vi "sequence1.vi"() -> ()   [LabVIEW 2021]
panel:
  out "Array":i64[](array[numeric])
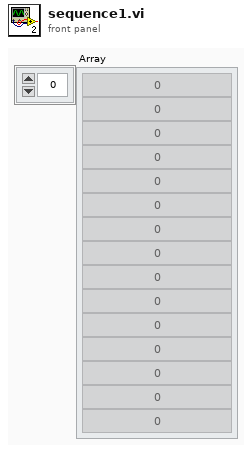
[diagram p1: front panel]
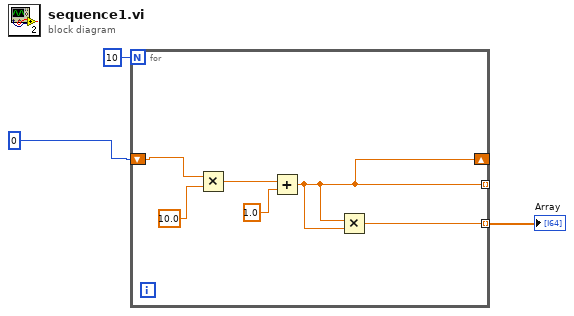
[diagram p0: block diagram]
diagram:
  n1 = for {
    N: 10 -> [_]
    shift-right: [w4] -> _
    shift-left: 0 -> [w8]
    tunnel: [w4] -> _ mode=indexing
    tunnel: [w6] -> w2 mode=indexing
    n2 = Multiply(x=w8, y=10.0) -> (x*y=w5:dbl)
    n3 = Add(x=w5, y=1.0) -> (x+y=w4:dbl)
    n4 = Multiply(x=w4, y=w4) -> (x*y=w6:dbl)
  }
  "Array" <- w2
